vi "Init_XE1000Pump.vi"(3 "XE 1000 Pump":refnum<visa-resource-name>="COM5") -> (0 "Connection":bool, 1 "XE 1000 Pump":refnum<visa-resource-name>)   [LabVIEW 2019]
uses:
  <vilib>/Instr/_visa.llb/VISA Configure Serial Port (Instr).vi
panel:
  in  "error in (no error)":errorcluster
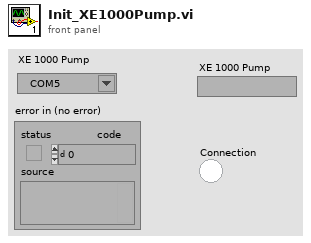
[diagram p1: front panel]
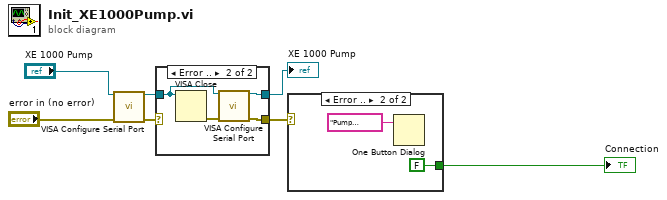
[diagram p0: block diagram]
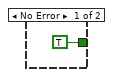
[diagram p2: hidden frame]
diagram:
  n1 = call-poly "VISA Configure Serial Port"("VISA resource name"="XE 1000 Pump", "error in (no error)"="error in (no error)") -> ("VISA resource name out"=w1:refnum<visa-resource-name>, "error out"=w6:errorcluster)  [unwired: 12 in]
  n2 = case shown="Error .." w6 {
    selector: w6 -> [w9 _]
    tunnel: [w9 w12] -> w3
    tunnel: w1 -> [w8 w13]
    tunnel: [w8 w11] -> w4
    frame No Error {
    }
    frame Error {
      n3 = VISA Close(VISA resource name=w13) -> (error out=w10:errorcluster)  [unwired: 1 in]
      n4 = call-poly "VISA Configure Serial Port"("VISA resource name"=w13, "error in (no error)"=w10) -> ("VISA resource name out"=w11:refnum<visa-resource-name>, "error out"=w12:errorcluster)  [unwired: 12 in]
    }
  }
  "XE 1000 Pump" <- w4
  n5 = case shown="Error .." w3 {
    tunnel: [TRUE FALSE] -> w2
    frame No Error {
    }
    frame Error {
      n6 = One Button Dialog(message="Pump connection error") -> ()  [unwired: 1 in, 1 out]
    }
  }
  "Connection" <- w2
